vi "Deg2Rad.vi"(1 "Input":dbl=1.0 min=-40.0 max=40.0 step=5.0 format="%.2f") -> (0 "Output":dbl=1.0 min=-40.0 max=40.0 step=5.0 format="%.2f")   [LabVIEW 2022 SP3]
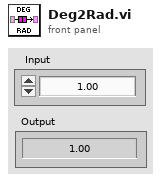
[diagram p1: front panel]
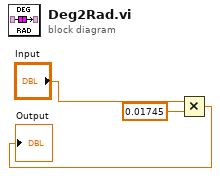
[diagram p0: block diagram]
diagram:
  n1 = Multiply(x="Input", y=0.01745) -> (x*y=→"Output":dbl)
